vi "Main.vi"() -> ()   [LabVIEW 2020]
doc: "This template is for the Queued Message Handler design pattern.\n\nThe Event Handling Loop generates messages based on user interface actions.\n\nThe Message Handling Loop processes messages generated by the Event Handling Loop, or by other messages. The messages are string values, so new messages can be added easily to the Message Cases case structure in the Message Handling Loop. Each message cluster can also provide an optional value for Message Data, which is a variant that can be converted to whatever message-specific data is required."
uses:
  controls/UI Data.ctl
  support/Message Queue/Message Cluster.ctl
  <extravilib>/ChannelInstances/Messenger-t'Message Queue.lvlib-Message Cluster.ctl'/Write With Abort.vi
  <extravilib>/ChannelInstances/Messenger-t'Message Queue.lvlib-Message Cluster.ctl'/Instantiate.vi
  <extravilib>/ChannelInstances/Messenger-t'Message Queue.lvlib-Message Cluster.ctl'/Endpoint.vi
  <extravilib>/ChannelInstances/Event Messenger-bool/Instantiate.vi
  <extravilib>/ChannelInstances/Event Messenger-bool/))Channel.vi
  <vilib>/Utility/error.llb/Error Cluster From Error Code.vi
  <vilib>/ErrorRing/Error Ring.xnode
  <extravilib>/ChannelInstances/Event Messenger-bool.lvlib
  support/Message Queue/Message Queue.lvlib
  <extravilib>/ChannelInstances/Messenger-t'Message Queue.lvlib-Message Cluster.ctl'.lvlib
panel:
  out "Display <Replace Me>":string
  in  "Do Something Else <Replace Me>":bool
  in  "Do Something <Replace Me>":bool
  in  "Exit":bool
  # "These controls have associated \"Value Changed\" events configured in the Event Structure on the diagram.\n\nReplace them (and reconfigure the Event Structure) with the controls you need for your application."
  # "This template is for the Queued Message Handler design pattern.\n\nSee the block diagram for more information on how to use this template."
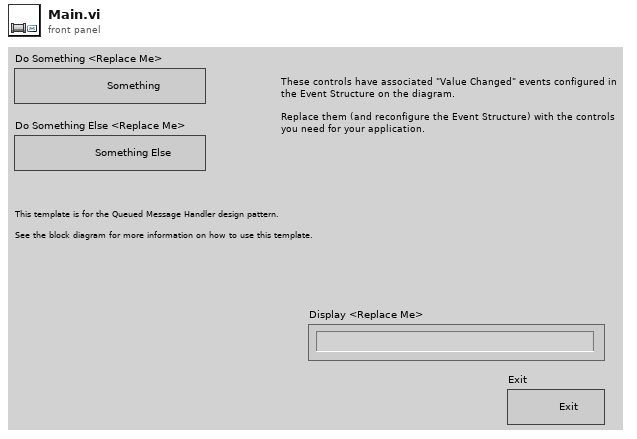
[diagram p1: front panel]
types:
  T1 = typedef "Message Queue.lvlib/Message Cluster.ctl" = cluster{"Message":string, "Message Data":variant}
  T2 = typedef "UI Data.ctl" = cluster{"String <Replace Me>":string, "Numeric <Replace Me>":u32}
  T3 = typedef "Messenger-t'Message Queue.lvlib-Message Cluster.ctl'.lvlib/))Channel.ctl" = refnum<queue>
  T4 = typedef "Event Messenger-bool.lvlib/))Channel.ctl" = refnum<queue>
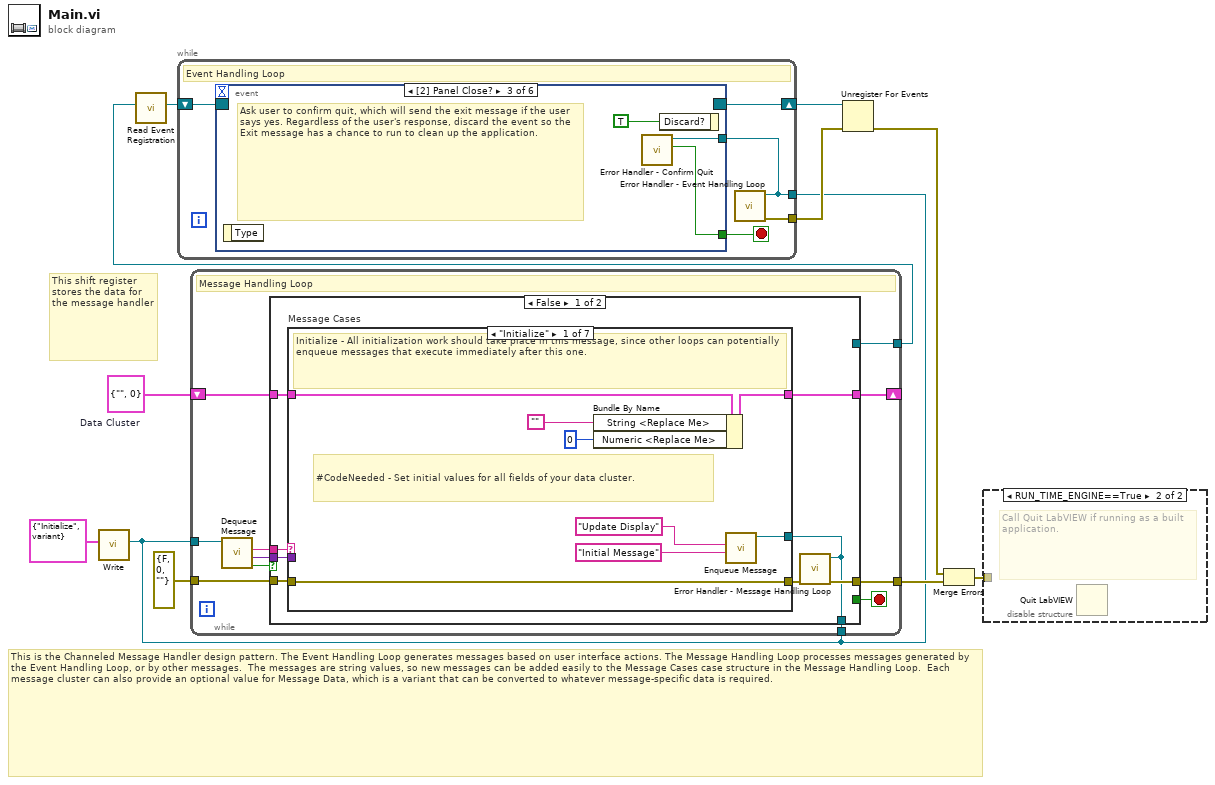
[diagram p0: block diagram]
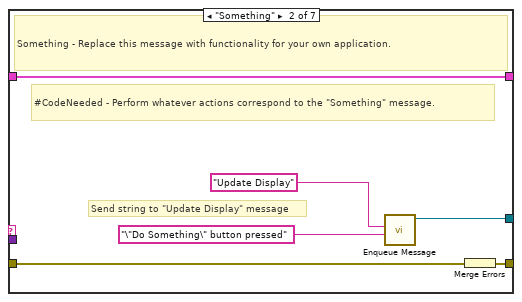
[diagram p2: hidden frame]
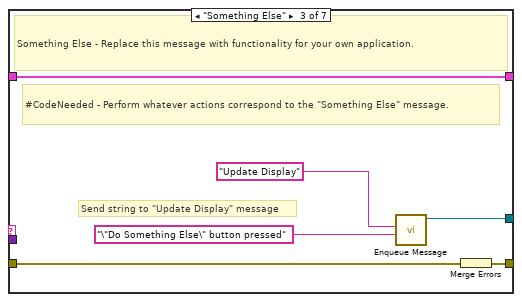
[diagram p3: hidden frame]
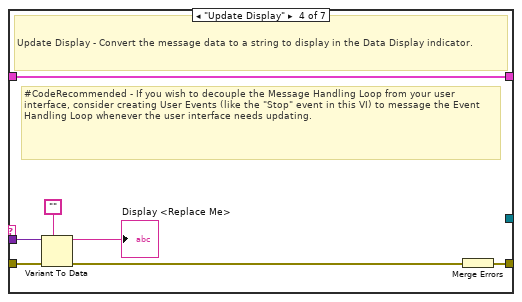
[diagram p4: hidden frame]
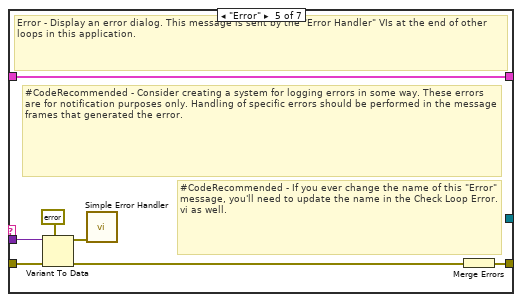
[diagram p5: hidden frame]
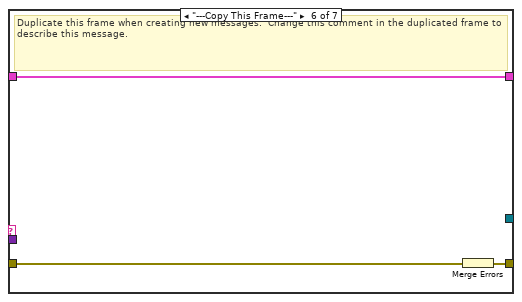
[diagram p6: hidden frame]
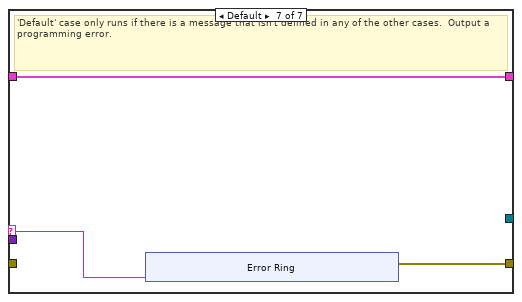
[diagram p7: hidden frame]
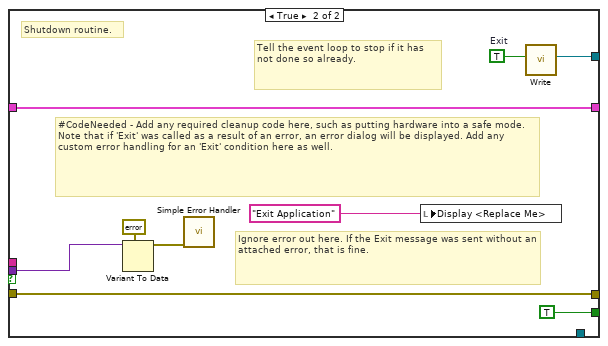
[diagram p8: hidden frame]
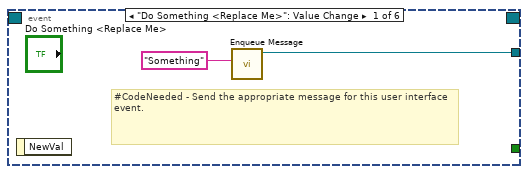
[diagram p10: hidden frame]
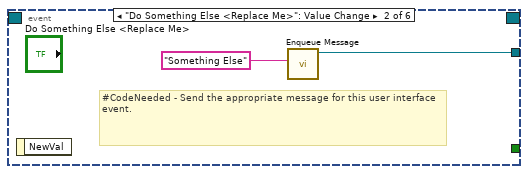
[diagram p11: hidden frame]
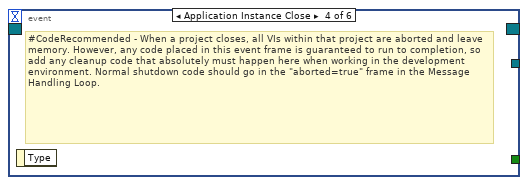
[diagram p12: hidden frame]
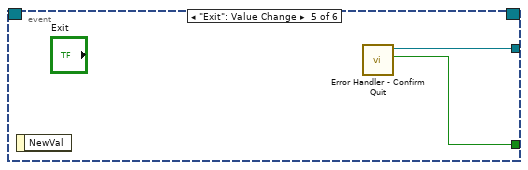
[diagram p13: hidden frame]
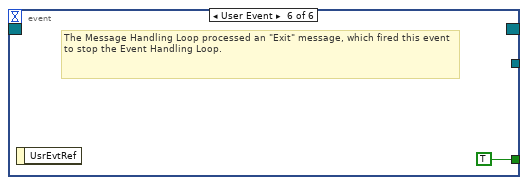
[diagram p14: hidden frame]
diagram:
  w8 = T2 {"String <Replace Me>"="", "Numeric <Replace Me>"=0}  # Data Cluster
  # "This is the Channeled Message Handler design pattern. The Event Handling Loop generates messages based on user interface actions. The Message Handling Loop processes messages generated by the Event Handling Loop, or by other messages.  The messages are string values, so new messages can be added easily to the Message Cases case structure in the Message Handling Loop.  Each message cluster can also provide an optional value for Message Data, which is a variant that can be converted to whatever message-specific data is required."
  # "This shift register stores the data for the message handler"
  n1 = call <extravilib>:"Write.vi"("element"=T1 {"Message"="Initialize", "Message Data"=variant}) -> ("channel"=w2:T3)  [unwired: 8 in, 2 out]
  n2 = while {
    shift-right: [w21] -> _
    shift-left: w8 -> [w22]
    tunnel: [w19] -> w11
    tunnel: [w18] -> w6
    tunnel: w2 -> [w15]
    tunnel: errorcluster {"status"=FALSE, "code"=0, "source"=""} ("error IO") -> [w17]
    tunnel: w2 -> [w16]
    stop <- w20 stop-if-true
    # "Message Handling Loop"
    n3 = call "Dequeue Message.vi"("channel"=w15) -> ("channel aborted"=w12:bool, "message data"=w13:variant, "message"=w14:string)  [unwired: 8 in]
    n4 = case shown="False" w12 {
      tunnel: w22 -> [w30 w84]
      tunnel: [w29 w84] -> w21
      tunnel: [_ TRUE] -> w20
      tunnel: [w28 w85] -> w19
      tunnel: [_ w79] -> w18
      tunnel: w14 -> [w26 _]
      tunnel: w13 -> [w25 w81]
      tunnel: w17 -> [w24 w85]
      tunnel: [w23 _] -> w16
      frame False {
        n5 = case "Message Cases" shown="\"Initialize\"" w26 {
          selector: w26 -> [_ _ _ _ _ _ w68]
          tunnel: w24 -> [w36 w42 w48 w55 w64 w67 _]
          tunnel: [w36 w43 w49 w56 w58 w65 w69] -> w27
          tunnel: w30 -> [w38 w44 w50 w57 w63 w66 w70]
          tunnel: [w37 w44 w50 w57 w63 w66 w70] -> w29
          tunnel: w25 -> [_ _ _ w54 w62 _ _]
          tunnel: [w33 w41 w47 _ _ _ _] -> w23
          frame "Initialize" {
            # "#CodeNeeded - Set initial values for all fields of your data cluster."
            # "Initialize - All initialization work should take place in this message, since other loops can potentially enqueue messages that execute immediately after this one."
            n6 = Bundle By Name(cluster=w38, "String <Replace Me>"="", "Numeric <Replace Me>"=u32 0) -> (w37:T2)
            n7 = call "Enqueue Message.vi"("data (empty)"="Initial Message" ("Initial Message"), "message"="Update Display" ("Message")) -> ("channel"=w33:T3)  [unwired: 9 in]
          }
          frame "Something" {
            # "Send string to \"Update Display\" message"
            # "#CodeNeeded - Perform whatever actions correspond to the \"Something\" message."
            # "Something - Replace this message with functionality for your own application."
            n8 = call "Enqueue Message.vi"("data (empty)"="\"Do Something\" button pressed" ("\"Do Something\" button pressed"), "message"="Update Display" ("Message")) -> ("channel"=w41:T3)  [unwired: 9 in]
            n9 = Merge Errors(w42) -> (w43:errorcluster)
          }
          frame "Something Else" {
            # "Send string to \"Update Display\" message"
            # "#CodeNeeded - Perform whatever actions correspond to the \"Something Else\" message."
            # "Something Else - Replace this message with functionality for your own application."
            n10 = call "Enqueue Message.vi"("data (empty)"="\"Do Something Else\" button pressed" ("\"Do Something Else\" button pressed"), "message"="Update Display" ("Message")) -> ("channel"=w47:T3)  [unwired: 9 in]
            n11 = Merge Errors(w48) -> (w49:errorcluster)
          }
          frame "Update Display" {
            # "#CodeRecommended - If you wish to decouple the Message Handling Loop from your user interface, consider creating User Events (like the \"Stop\" event in this VI) to message the Event Handling Loop whenever the user interface needs updating."
            # "Update Display - Convert the message data to a string to display in the Data Display indicator."
            n12 = Variant To Data(error in=w55, type="", Variant=w54) -> (data=→"Display <Replace Me>":string, error out=w52:errorcluster)
            n13 = Merge Errors(w52) -> (w56:errorcluster)
          }
          frame "Error" {
            # "#CodeRecommended - If you ever change the name of this \"Error\" message, you'll need to update the name in the Check Loop Error.vi as well."
            # "#CodeRecommended - Consider creating a system for logging errors in some way. These errors are for notification purposes only. Handling of specific errors should be performed in the message frames that generated the error."
            # "Error - Display an error dialog. This message is sent by the \"Error Handler\" VIs at the end of other loops in this application."
            n14 = Variant To Data(error in=w64, type=errorcluster {"status"=FALSE, "code"=0, "source"=""} ("error constant"), Variant=w62) -> (data=w60:errorcluster, error out=w59:errorcluster)
            n15 = call <vilib>:"Simple Error Handler.vi"("error in (no error)"=w60) -> ()  [unwired: 4 in, 5 out]
            n16 = Merge Errors(w59) -> (w58:errorcluster)
          }
          frame "---Copy This Frame---" {
            # "Duplicate this frame when creating new messages.  Change this comment in the duplicated frame to describe this message."
            n17 = Merge Errors(w67) -> (w65:errorcluster)
          }
          frame Default {
            # "'Default' case only runs if there is a message that isn't defined in any of the other cases.  Output a programming error."
            n18 = xnode "Error Ring"("parameter 0"=w68) -> ("error out"=w69:errorcluster)
          }
        }
        n19 = call "Error Handler - Message Handling Loop.vi"("channel"=w23, "error in (no error)"=w27) -> ("dup error in"=w28:errorcluster)  [unwired: 9 in]
      }
      frame True {
        w80 = TRUE  # Exit
        # "Tell the event loop to stop if it has not done so already."
        # "Ignore error out here. If the Exit message was sent without an attached error, that is fine."
        # "#CodeNeeded - Add any required cleanup code here, such as putting hardware into a safe mode. Note that if 'Exit' was called as a result of an error, an error dialog will be displayed. Add any custom error handling for an 'Exit' condition here as well."
        # "Shutdown routine."
        n20 = Variant To Data(type=errorcluster {"status"=FALSE, "code"=0, "source"=""} ("error constant"), Variant=w81) -> (data=w82:errorcluster)  [unwired: 1 in, 1 out]
        n21 = call <vilib>:"Simple Error Handler.vi"("error in (no error)"=w82) -> ()  [unwired: 4 in, 5 out]
        n22 = local write "Display <Replace Me>"("Exit Application" ("Exit Application")) -> ()
        n23 = call <extravilib>:"Write.vi"("element"=w80) -> ("channel"=w79:T4)  [unwired: 9 in, 1 out]
      }
    }
  }
  n24 = call <extravilib>:"Read Event Registration.vi"("channel"=w6) -> ("event registration refnum"=w5:refnum<event-registration>)  [unwired: 10 in]
  n25 = while {
    shift-right: [w90] -> w9
    shift-left: w5 -> [w91]
    tunnel: [w88] -> w7
    tunnel: w2 -> [w87]
    stop <- w89 stop-if-true
    # "Event Handling Loop"
    n26 = event shown="[2] Panel Close?" {
      selector: w91 -> [_ _ _ _ _ _]
      dyn-events: [_ _ _ _ _ _] -> w90
      timeout: _ -> [_ _ _ _ _ _]
      tunnel: [_ _ w96 _ w99 TRUE ("Discard?")] -> w89
      tunnel: [w93 w95 w97 _ w100 _] -> w87
      event "Do Something <Replace Me>": Value Change {
        # "#CodeNeeded - Send the appropriate message for this user interface event."
        n27 = event-data() -> ()  [unwired: 1 in, 1 out]
        n28 = call "Enqueue Message.vi"("message"="Something" ("Message")) -> ("channel"=w93:T3)  [unwired: 10 in]
      }
      event "Do Something Else <Replace Me>": Value Change {
        # "#CodeNeeded - Send the appropriate message for this user interface event."
        n29 = event-data() -> ()  [unwired: 1 in, 1 out]
        n30 = call "Enqueue Message.vi"("message"="Something Else" ("Message")) -> ("channel"=w95:T3)  [unwired: 10 in]
      }
      event Panel Close? {
        # "Ask user to confirm quit, which will send the exit message if the user says yes. Regardless of the user's response, discard the event so the Exit message has a chance to run to clean up the application."
        n31 = event-data() -> ()  [unwired: 1 in, 1 out]
        n32 = call "Error Handler - Confirm Quit.vi"() -> ("exit confirmed"=w96:bool, "channel"=w97:T3)  [unwired: 10 in]
        n33 = event-data("Discard?"=TRUE) -> ()  [unwired: 1 in, 1 out]
      }
      event Application Instance Close {
        # "#CodeRecommended - When a project closes, all VIs within that project are aborted and leave memory. However, any code placed in this event frame is guaranteed to run to completion, so add any cleanup code that absolutely must happen here when working in the development environment. Normal shutdown code should go in the \"aborted=true\" frame in the Message Handling Loop."
        n34 = event-data() -> ()  [unwired: 1 in, 1 out]
      }
      event "Exit": Value Change {
        n35 = event-data() -> ()  [unwired: 1 in, 1 out]
        n36 = call "Error Handler - Confirm Quit.vi"() -> ("exit confirmed"=w99:bool, "channel"=w100:T3)  [unwired: 10 in]
      }
      event User Event {
        # "The Message Handling Loop processed an \"Exit\" message, which fired this event to stop the Event Handling Loop."
        n37 = event-data() -> ()  [unwired: 1 in, 1 out]
      }
    }
    n38 = call "Error Handler - Event Handling Loop.vi"("channel"=w87) -> ("dup error in"=w88:errorcluster)  [unwired: 10 in]
  }
  n39 = Unregister For Events(event registration refnum=w9, error in=w7) -> (error out=w10:errorcluster)
  n40 = Merge Errors(w10, w11) -> (w4:errorcluster)
  n41 = disable-structure shown="RUN_TIME_ENGINE==True" {
    disable-tunnel: w4 -> [_ _]
    frame condition #0 (active) {
    }
    frame condition #1 {
      # "Call Quit LabVIEW if running as a built application."
      n42 = Quit LabVIEW() -> ()  [unwired: 1 in]
    }
  }
